vi "OSICS_Get_Mode_SWT-APC.vi"(7 "OSICS slot":i32=1 min=1 max=8 step=1, 8 "error in":errorcluster, 11 "VISA IN":refnum<visa-resource-name>) -> (0 "error out":errorcluster, 2 "Mode setting":string, 3 "VISA OUT":refnum<visa-resource-name>, 5 "ERR":i32)   [LabVIEW 2014, in "OSICS_LIB.lvlib"]
doc: "This Vi request the operating mode of the OSICS module SWT-APC."
uses:
  OSICS_LIB.lvlib
panel:
  # "Basic Function to set the power units and power output\nfor the OSICS"
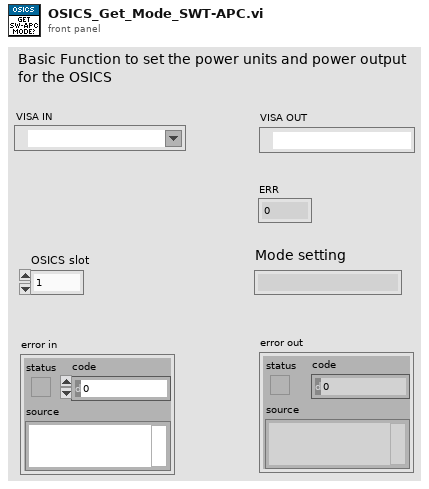
[diagram p1: front panel]
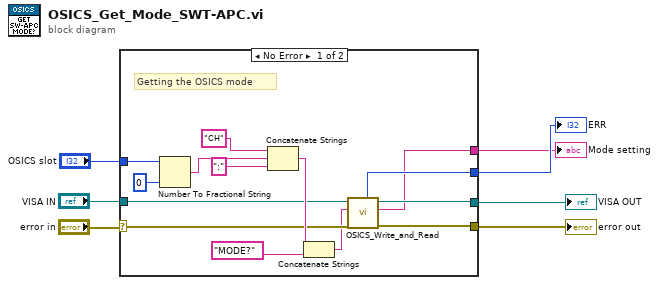
[diagram p0: block diagram]
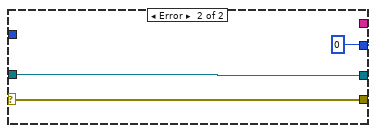
[diagram p2: hidden frame]
diagram:
  n1 = case shown="No Error" "error in" {
    selector: "error in" -> [w15 w23]
    tunnel: "VISA IN" -> [w14 w24]
    tunnel: [w11 w24] -> w6
    tunnel: [w10 w23] -> w5
    tunnel: [w12 0 ("ERR")] -> w3
    tunnel: "OSICS slot" -> [w21 _]
    tunnel: [w8 _] -> w1
    frame No Error {
      # "Getting the OSICS mode"
      n2 = Number To Fractional String(number=w21, precision (6)=i16 0) -> (F-format string=w18:string)  [unwired: 2 in]
      n3 = Concatenate Strings("CH" ("string"), w18, ":" ("string")) -> (w16:string)
      n4 = Concatenate Strings(w16, "MODE?" ("string")) -> (w13:string)
      n5 = call "OSICS_Write_and_Read.vi"("error in (no error)"=w15, "String to Send"=w13, "VISA IN"=w14) -> ("error out"=w10:errorcluster, "Message Available"=w8:string, "VISA OUT"=w11:refnum<visa-resource-name>, "ERR"=w12:i32)  [unwired: 5 in]
    }
    frame Error {
    }
  }
  "error out" <- w5
  "VISA OUT" <- w6
  "ERR" <- w3
  "Mode setting" <- w1
